vi "ReadBuffers.vi"(8 "Error In":errorcluster, 10 "Measure Configurations":T1[](array[typedef]) {"Count" min=1 step=1}, 11 "Kiethley 2602 In":refnum<visa-resource-name>) -> (0 "Error Out":errorcluster, 2 "Data":dbl[][](array[numeric]), 3 "Keithley 2602 Out":refnum<visa-resource-name>)   [LabVIEW 2012]
uses:
  MeasureConfiguration.ctl
  driver/Public/Controls/SMU.ctl
  driver/Keithley-2602.lvlib
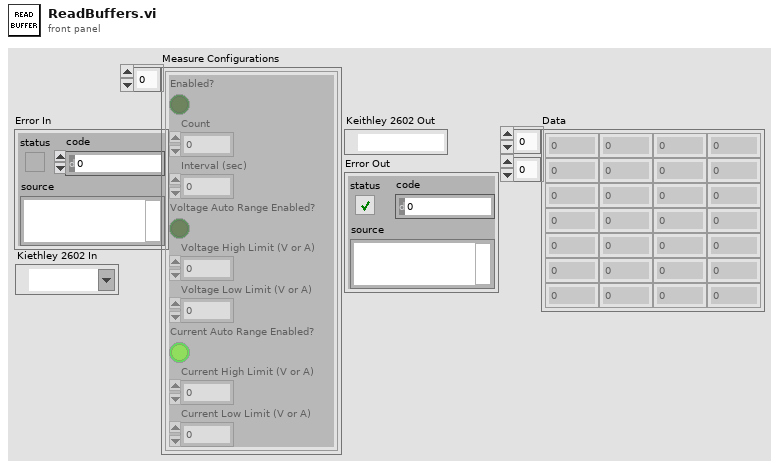
[diagram p1: front panel]
types:
  T1 = typedef "MeasureConfiguration.ctl" = cluster{"Enabled?":bool, "Count":u8, "Interval (sec)":dbl, "Voltage Auto Range Enabled?":bool, "Voltage High Limit (V or A)":dbl, "Voltage Low Limit (V or A)":dbl, "Current Auto Range Enabled?":bool, "Current High Limit (V or A)":dbl, "Current Low Limit (V or A)":dbl}
  T2 = typedef "Keithley-2602.lvlib/SMU.ctl" = enum16{"A", "B"}
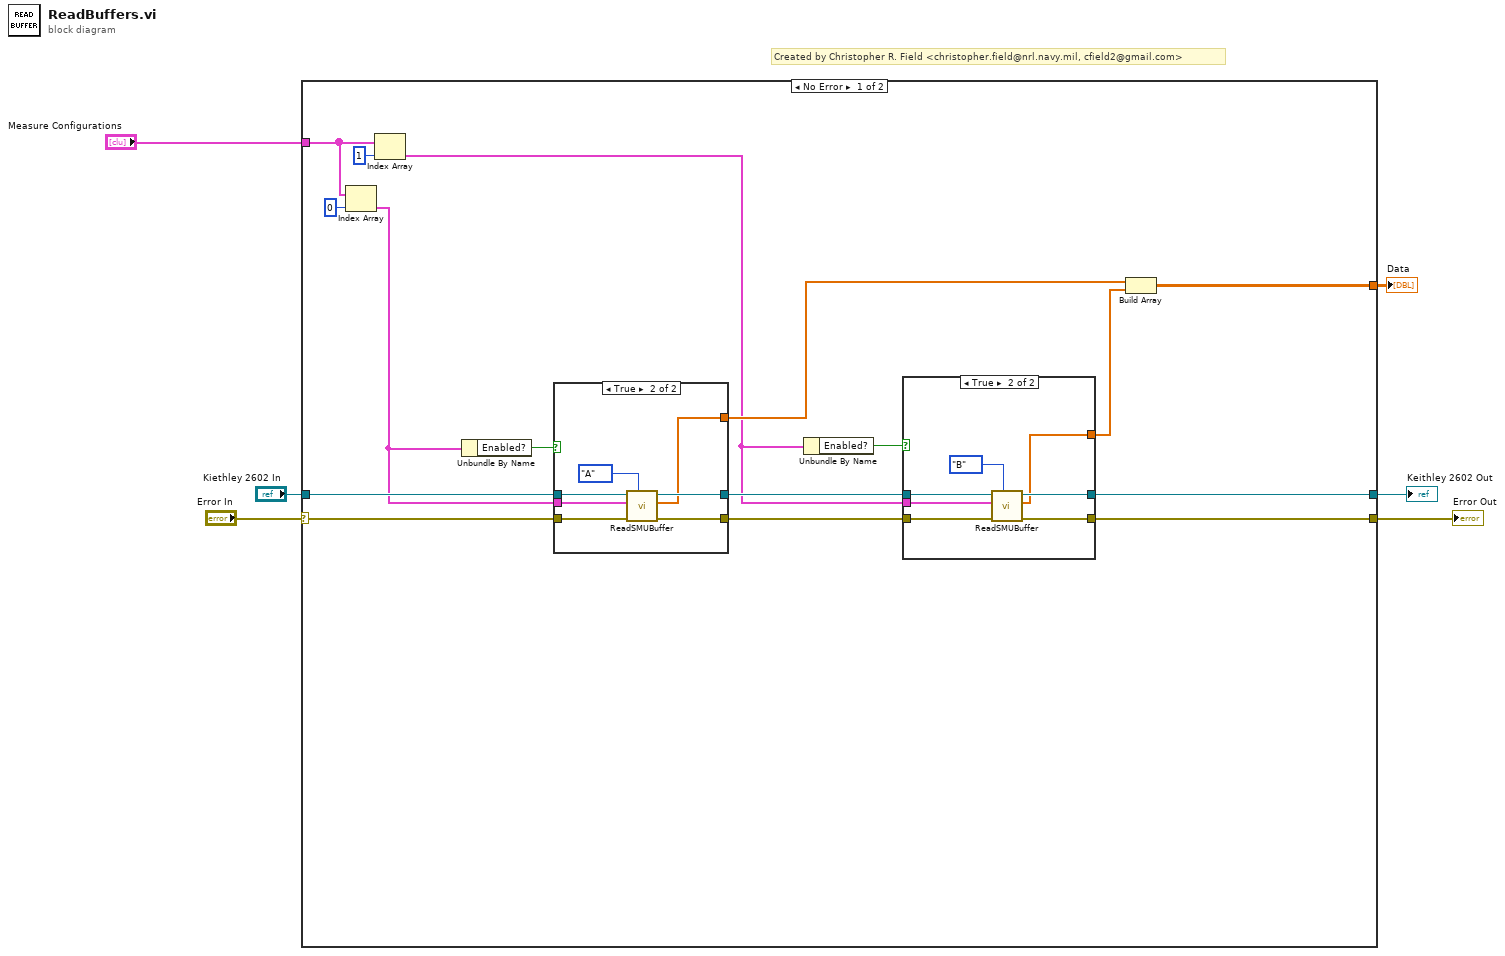
[diagram p0: block diagram]
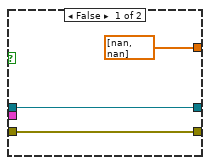
[diagram p2: hidden frame]
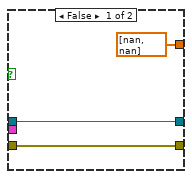
[diagram p3: hidden frame]
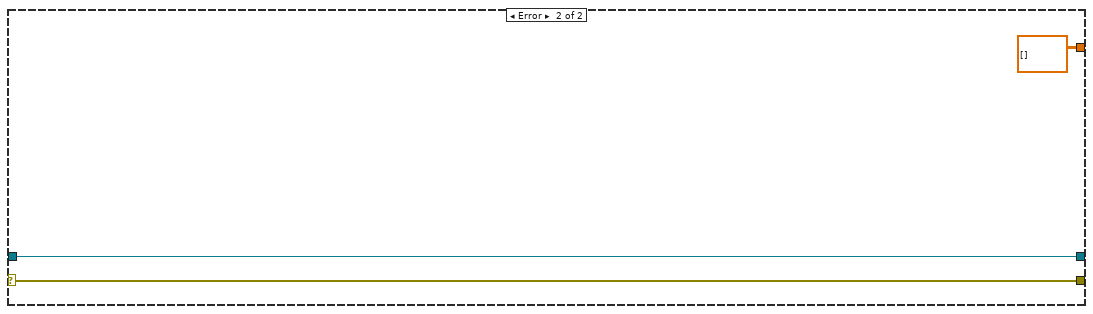
[diagram p4: hidden frame]
diagram:
  # "Created by Christopher R. Field <christopher.field@nrl.navy.mil, cfield2@gmail.com>"
  n1 = case shown="No Error" "Error In" {
    selector: "Error In" -> [w21 w44]
    tunnel: "Kiethley 2602 In" -> [w22 w45]
    tunnel: [w18 w45] -> w4
    tunnel: [w17 w44] -> w3
    tunnel: [w9 dbl[][] []] -> w2
    tunnel: "Measure Configurations" -> [w13 _]
    frame No Error {
      n2 = Index Array(array=w13, index=0) -> (element=w7:T1)
      n3 = Index Array(array=w13, index=1) -> (element=w8:T1)
      n4 = Unbundle By Name(w7) -> ("Enabled?"=w12:bool)
      n5 = case shown="True" w12 {
        tunnel: w22 -> [w35 w42]
        tunnel: w21 -> [w34 w41]
        tunnel: [w35 w39] -> w20
        tunnel: [w34 w38] -> w19
        tunnel: w7 -> [_ w37]
        tunnel: [dbl[] [nan, nan] ("Data") w36] -> w11
        frame False {
        }
        frame True {
          n6 = call "ReadSMUBuffer.vi"("SMU"=SMU."A", "Error In"=w41, "Measure Configuration"=w37, "Kiethley 2602 In"=w42) -> ("Error Out"=w38:errorcluster, "Data"=w36:dbl[], "Keithley 2602 Out"=w39:refnum<visa-resource-name>)  [unwired: 5 in]
        }
      }
      n7 = Unbundle By Name(w8) -> ("Enabled?"=w15:bool)
      n8 = case shown="True" w15 {
        tunnel: w20 -> [w25 w32]
        tunnel: w19 -> [w24 w31]
        tunnel: [w25 w29] -> w18
        tunnel: [w24 w28] -> w17
        tunnel: w8 -> [_ w27]
        tunnel: [dbl[] [nan, nan] ("Data") w26] -> w10
        frame False {
        }
        frame True {
          n9 = call "ReadSMUBuffer.vi"("SMU"=SMU."B", "Error In"=w31, "Measure Configuration"=w27, "Kiethley 2602 In"=w32) -> ("Error Out"=w28:errorcluster, "Data"=w26:dbl[], "Keithley 2602 Out"=w29:refnum<visa-resource-name>)  [unwired: 5 in]
        }
      }
      n10 = Build Array(w11, w10) -> (w9:dbl[][])
    }
    frame Error {
    }
  }
  "Keithley 2602 Out" <- w4
  "Error Out" <- w3
  "Data" <- w2
